vi "Filter Line ROIContours.vi"(8 "error in (no error)":errorcluster, 11 "Analyze BaseClass in":refnum<class "Analyze BaseClass.lvclass">) -> (0 "error out":errorcluster, 2 "Line contours":T1 {"Contours"."Type" items=["No Selection", "Point", "Line", "Rectangle", "Oval", "Polygon", "Freehand Region", "Annulus", "Unused2", "Unused3", "Broken Line", "Freehand Line", "Rotated Rectangle"]}, 3 "Analyze BaseClass out":refnum<class "Analyze BaseClass.lvclass">)   [LabVIEW 2014, in "Analyze.lvlib" / "Analyze BaseClass.lvlib" / "Analyze BaseClass.lvclass"]
uses:
  Analyze BaseClass.lvclass
  Analyze Parameter/Analyze Parameter ROI/Analyze Parameter ROI.lvclass
  Analyze Parameter/Analyze Parameter ROI/Analyze Parameter ROI.lvclass/Analyze Parameter ROI.ctl
  Analyze Parameter/Analyze Parameter ROI/Read ROI Descriptor.vi
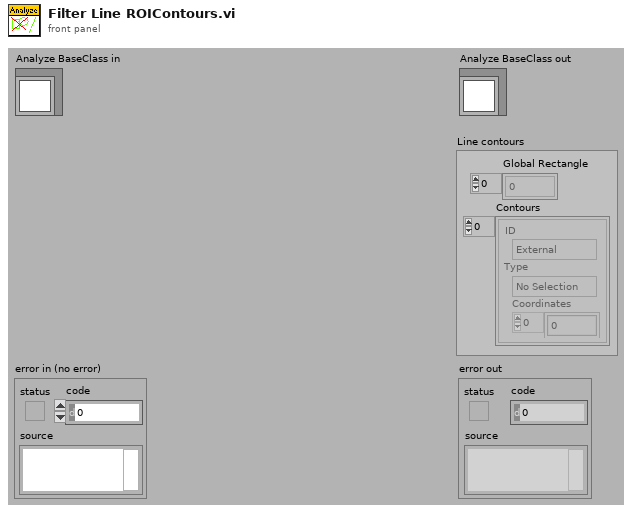
[diagram p1: front panel]
types:
  T1 = typedef "ROI Descriptor" = cluster{"Global Rectangle":i32[], "Contours":cluster{"ID":enum32{"External", "Internal"}, "Type":u32, "Coordinates":i32[]}[]}
  T2 = cluster{"ID":enum32{"External", "Internal"}, "Type":u32, "Coordinates":i32[]}[]
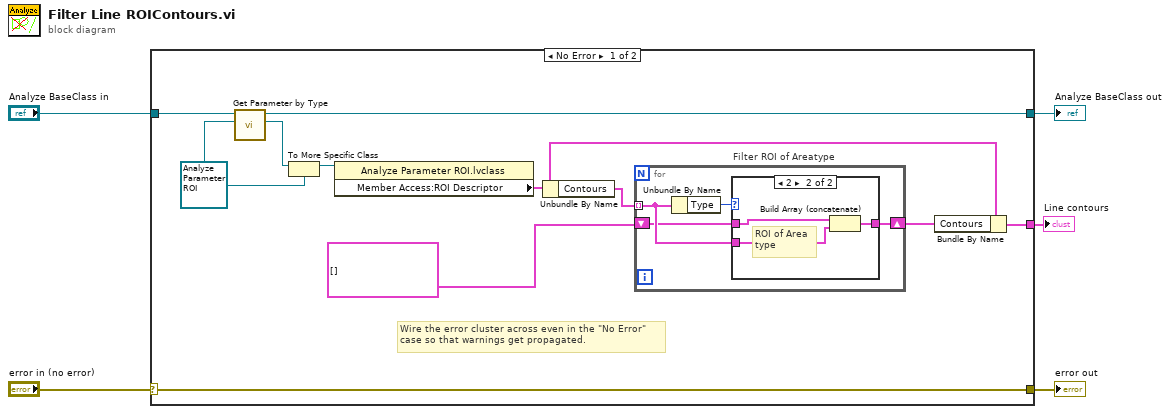
[diagram p0: block diagram]
diagram:
  n1 = case shown="No Error" "error in (no error)" {
    selector: "error in (no error)" -> [w16 w26]
    tunnel: [w16 w26] -> w4
    tunnel: [w9 w25] -> w2
    tunnel: "Analyze BaseClass in" -> [w10 w25]
    tunnel: [w13 _] -> w1
    frame No Error {
      w8 = refnum<class "Analyze Parameter ROI.lvclass"> refnum ("Analyze Parameter ROI.lvclass")
      # "Wire the error cluster across even in the \"No Error\"\ncase so that warnings get propagated."
      n2 = call "Get Parameter by Type.vi"("Parameter Type"=w8, "Analyze BaseClass in"=w10) -> ("Parameter"=w7:refnum<class "Analyze Parameter Base.lvclass">, "Analyze BaseClass out"=w9:refnum<class "Analyze BaseClass.lvclass">)  [unwired: 6 in, 2 out]
      n3 = To More Specific Class(target class=w8, reference=w7) -> (specific class reference=w6:refnum<class "Analyze Parameter ROI.lvclass">)  [unwired: 1 in, 1 out]
      n4 = property class="Analyze Parameter ROI.lvclass"(reference=w6) -> ("Member Access:ROI Descriptor"=w11:T1)  [unwired: 1 in, 2 out]
      n5 = Unbundle By Name(w11) -> ("Contours"=w12:T2)
      n6 = for "Filter ROI of Areatype" {
        tunnel: w12 -> [w19] mode=indexing
        shift-right: [w18] -> w14
        shift-left: T2 [] -> [w17]
        n7 = Unbundle By Name(w19) -> ("Type"=w20:u32)
        n8 = case shown="2" w20 {
          tunnel: w19 -> [_ w24]
          tunnel: [w21 w23] -> w18
          tunnel: w17 -> [w21 w22]
          frame 0, Default {
          }
          frame 2 {
            # "ROI of Area\ntype"
            n9 = Build Array (concatenate)(w22, w24) -> (w23:T2)
          }
        }
      }
      n10 = Bundle By Name(cluster=w11, "Contours"=w14) -> (w13:T1)
    }
    frame Error {
    }
  }
  "error out" <- w4
  "Analyze BaseClass out" <- w2
  "Line contours" <- w1
